vi "File.Filter Subdirectories by Name.vi"(10 "From_To":string[](array[string]), 11 "RootDir":path) -> (3 "SubDirs":path[](array[path]))   [LabVIEW 2024]
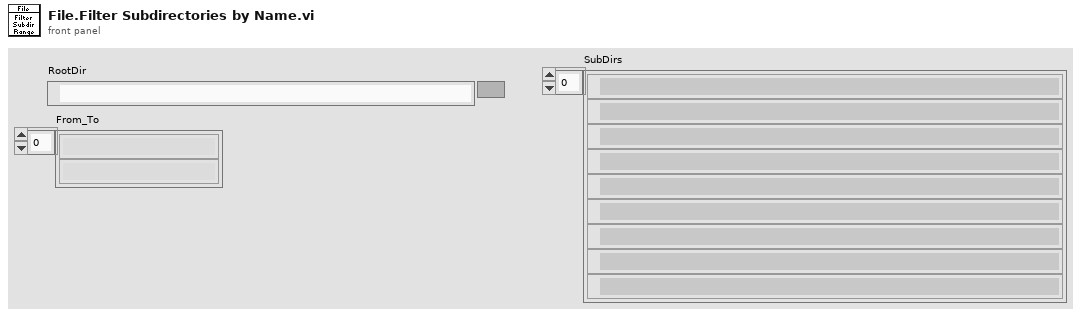
[diagram p1: front panel]
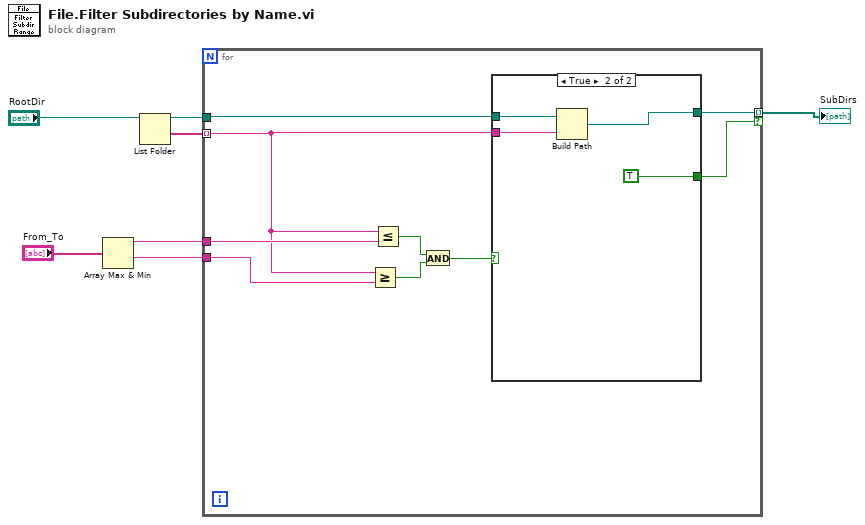
[diagram p0: block diagram]
diagram:
  n1 = Array Max & Min(array="From_To") -> (max value=w3:string, min value=w2:string)  [unwired: 2 out]
  n2 = List Folder(path="RootDir") -> (path out=w6:path, folder names=w5:string[])  [unwired: 3 in, 2 out]
  n3 = for {
    tunnel: w6 -> [w12]
    tunnel: w5 -> [w11] mode=indexing
    tunnel: w3 -> [w15]
    tunnel: w2 -> [w16]
    tunnel: [w9] -> w1 mode=indexing if=w8
    n4 = Greater Or Equal?(x=w11, y=w16) -> (x >= y?=w13:bool)
    n5 = Less Or Equal?(x=w11, y=w15) -> (x <= y?=w14:bool)
    n6 = And(x=w14, y=w13) -> (x .and. y?=w10:bool)
    n7 = case shown="True" w10 {
      tunnel: w12 -> [_ w20]
      tunnel: w11 -> [_ w19]
      tunnel: [_ w18] -> w9
      tunnel: [_ TRUE] -> w8
      frame False {
      }
      frame True {
        n8 = Build Path(base path=w20, name or relative path=w19) -> (appended path=w18:path)
      }
    }
  }
  "SubDirs" <- w1
